vi "sysparam.vi"() -> (1 "C":dbl[][](array[numeric]), 2 "K":dbl[][](array[numeric]), 3 "A":dbl[][](array[numeric]))   [LabVIEW 2015]
uses:
  <vilib>/imath/engines/lvmath2/RunTimeEngine/Managers/WorkSpace/UID Generator.vi
  <vilib>/imath/engines/lvmath2/RunTimeEngine/RunTimeType/NIMS_RunTimeType_From StrictType (excl LVString).vi
  <instcachedir>/0/NIMS_RunTimeType_From StrictType (excl LVString)_EB1C38A9BC5048DA9ABDA8F781E54D21.lvgen/NIMS_RunTimeType_From StrictType (excl LVString)_EB1C38A9BC5048DA9ABDA8F781E54D21_000.vi
  <vilib>/imath/engines/lvmath2/RunTimeEngine/LocalVariableDefStatement/MC_LocalVariableDefStatement_Display.vi
  <vilib>/imath/engines/lvmath2/RunTimeEngine/Managers/SymbolTable/Clear UID.vi
  <vilib>/imath/engines/lvmath2/RunTimeEngine/NodeEndStatement/NIMS_NodeEndStatement_Output.vi
  <instcachedir>/0/NIMS_NodeEndStatement_Output_53EC0D466D134D7ABD903AC30B43404B.lvgen/NIMS_NodeEndStatement_Output_53EC0D466D134D7ABD903AC30B43404B_010.vi
  <instcachedir>/0/NIMS_NodeEndStatement_Output_53EC0D466D134D7ABD903AC30B43404B.lvgen/NIMS_NodeEndStatement_Output_53EC0D466D134D7ABD903AC30B43404B_002.vi
  <vilib>/imath/engines/lvmath2/RunTimeEngine/ErrorHandling/NIMS_Finalize Error.vi
  <vilib>/imath/engines/lvmath2/RunTimeEngine/Managers/SymbolTable/NIMS_WorkSpace.lvlib
panel:
  in  "az":dbl=0.45
  in  "ay":dbl=0.45
  in  "ax":dbl=0.45
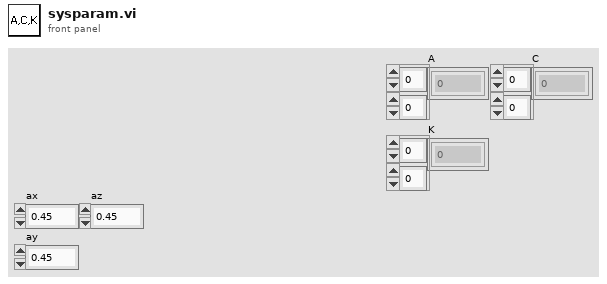
[diagram p1: front panel]
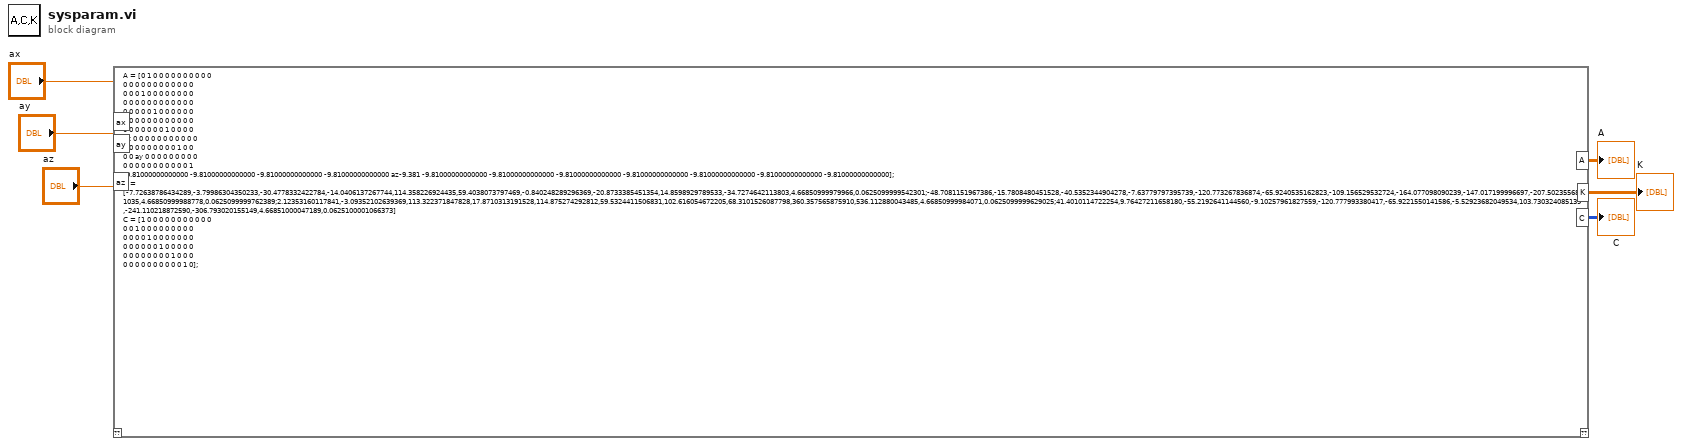
[diagram p0: block diagram]
diagram:
  n1 = mathscript code="A = [0\t1\t0\t0\t0\t0\t0\t0\t0\t0\t0\t0\n0\t0\t0\t0\t0\t0\t0\t0\t0\t0\t0\t0\n0\t0\t0\t1\t0\t0\t0\t0\t0\t0\t0\t0\n0\t0\t0\t0\t0\t0\t0\t0\t0\t0\t0\t0\n0\t0\t0\t0\t0\t1\t0\t0\t0\t0\t0\t0\n0\t0\t0\t0\t0\t0\t0\t0\t0\t0\t0\t0\n0\t0\t0\t0\t0\t0\t0\t1\t0\t0\t0\t0\nax\t0\t0\t0\t0\t0\t0\t0\t0\t0\t0\t0\n0\t0\t0\t0\t0\t0\t0\t0\t0\t1\t0\t0\n0\t0\tay\t0\t0\t0\t0\t0\t0\t0\t0\t0\n0\t0\t0\t0\t0\t0\t0\t0\t0\t0\t0\t1\n-9.81000000000000\t-9.81000000000000\t-9.81000000000000\t-9.81000000000000\taz-9.381\t-9.81000000000000\t-9.81000000000000\t-9.81000000000000\t-9.81000000000000\t-9.81000000000000\t-9.81000000000000\t-9.81000000000000];\nK = [-7.72638786434289,-3.79986304350233,-30.4778332422784,-14.0406137267744,114.358226924435,59.4038073797469,-0.840248289296369,-20.8733385451354,14.8598929789533,-34.7274642113803,4.66850999979966,0.0625099999542301;-48.7081151967386,-15.7808480451528,-40.5352344904278,-7.63779797395739,-120.773267836874,-65.9240535162823,-109.156529532724,-164.077098090239,-147.017199996697,-207.502355681035,4.66850999988778,0.0625099999762389;2.12353160117841,-3.09352102639369,113.322371847828,17.8710313191528,114.875274292812,59.5324411506831,102.616054672205,68.3101526087798,360.357565875910,536.112880043485,4.66850999984071,0.0625099999629025;41.4010114722254,9.76427211658180,-55.2192641144560,-9.10257961827559,-120.777993380417,-65.9221550141586,-5.52923682049534,103.730324085139,-241.110218872590,-306.793020155149,4.66851000047189,0.0625100001066373]\nC = [1\t0\t0\t0\t0\t0\t0\t0\t0\t0\t0\t0\n0\t0\t1\t0\t0\t0\t0\t0\t0\t0\t0\t0\n0\t0\t0\t0\t1\t0\t0\t0\t0\t0\t0\t0\n0\t0\t0\t0\t0\t0\t1\t0\t0\t0\t0\t0\n0\t0\t0\t0\t0\t0\t0\t0\t1\t0\t0\t0\n0\t0\t0\t0\t0\t0\t0\t0\t0\t0\t1\t0];"("ax"="ax", "ay"="ay", "az"="az") -> ("A"=→"A":dbl[][], "K"=→"K":dbl[][], "C"=→"C":i32[][])  [unwired: 1 in, 1 out]
